vi "ClimbGetSensorPoseRight.vi"() -> (0 "ClimbGetSensorPoseRight":dbl)   [LabVIEW 2023]
uses:
  ClimbGlobal.vi
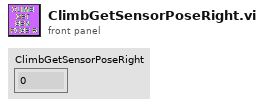
[diagram p1: front panel]
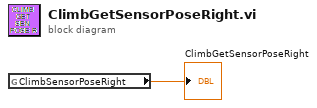
[diagram p0: block diagram]
diagram:
  n1 = global read "ClimbGlobal.vi" "ClimbSensorPoseRight"() -> (→"ClimbGetSensorPoseRight":dbl)
